vi "Write Local Resource.vi"(8 "error in (no error)":errorcluster, 10 "resource name":refnum<k15> caption="Local Resource", 11 "5105 in":refnum<class "5105.lvclass">) -> (0 "error out":errorcluster, 3 "5105 out":refnum<class "5105.lvclass">)   [LabVIEW 2019, in "5105.lvlib" / "5105.lvclass"]
uses:
  5105.lvclass
  5105.lvclass/5105.ctl
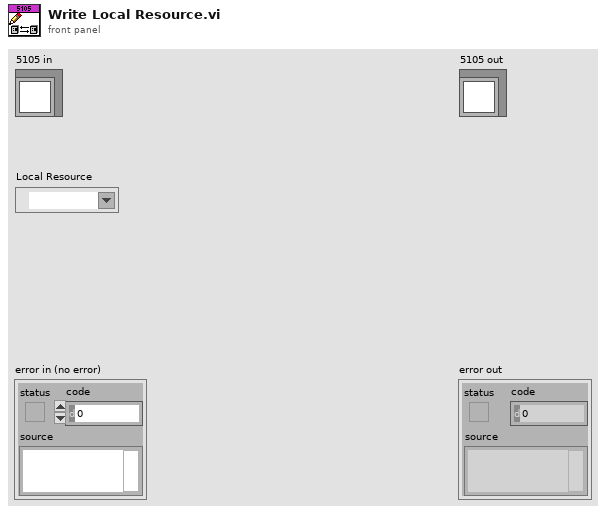
[diagram p1: front panel]
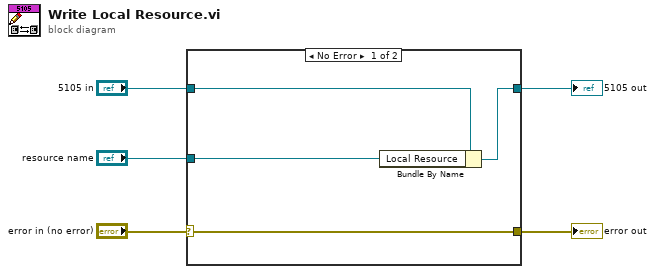
[diagram p0: block diagram]
diagram:
  n1 = case shown="No Error" "error in (no error)" {
    selector: "error in (no error)" -> [w6 w10]
    tunnel: "5105 in" -> [w9 w11]
    tunnel: "resource name" -> [w8 _]
    tunnel: [w7 w11] -> w1
    tunnel: [w6 w10] -> w2
    frame No Error {
      n2 = Bundle By Name(cluster=w9, "Local Resource"=w8) -> (w7:refnum<class "5105.lvclass">)
    }
    frame Error {
    }
  }
  "error out" <- w2
  "5105 out" <- w1
